vi "Set G08 Delay.vi"(7 "DG Number":i32, 8 "error in (no error)":errorcluster, 11 "Settings":T1={"Channel"=2, "Fire First (µs)"=0.0, "Pulse Width (µs)"=0.005, "Output Modulo"=1, "Output Offset"=0, "Go Signal"=16, "Polarity"=TRUE, "Terminate"=TRUE, "Disconnect (E,F)"=FALSE, "Onto MsBus (E,F)"=FALSE, "Input Positive (E,F)"=TRUE} {"Go Signal" format="%04x" items=["Local Primary"=1, "Local Secondary"=2, "Local Force"=4, "Resynchronize"=8, "Master Primary"=16, "Master Secondary"=32, "Master Force"=64, "System Clock"=128, "Delay Clock"=256, "Inhibit Local"=512, "Start Local"=1024, "Start Bus"=2048, "Step Back Local"=4096, "Step Back Bus"=8192, "From E"=65536, "From F"=131072, "From Bus"=262144]; "Pulse Width (µs)" min=0.0 max=8947840.0 format="%.6f"; "Fire First (µs)" min=0.0 format="%.6f"; "Channel" items=["T"=1, "A"=2, "B"=3, "C"=4, "D"=5, "E"=6, "F"=7]}) -> (0 "error out":errorcluster)   [LabVIEW 2009, in "POLARIS BME DG.lvlib"]
doc: "long Set_BME_G05(double FireFirst_T0, unsigned long OutputModulo_T0, BOOL Active_T0, BOOL Positive_T0, BOOL Terminate_T0, BOOL HighDrive_T0, double FireFirst_A, unsigned long OutputModulo_A, BOOL Active_A, BOOL Positive_A, BOOL Terminate_A, BOOL HighDrive_A, double FireFirst_B, unsigned long OutputModulo_B, BOOL Active_B, BOOL Positive_B, BOOL Terminate_B, BOOL HighDrive_B, BOOL Gate_AB, unsigned long OutputLevel, BOOL TriggerTerminate, BOOL ClockEnable, double InternalClock, double TriggerLevel, unsigned long PresetValue, unsigned long DivideBy, unsigned long ClockSource, unsigned long GateDivider, BOOL PositiveGate, BOOL InternalTrigger, BOOL InternalArm, BOOL SoftwareTrigger, BOOL RisingEdge, BOOL StopOnPreset, BOOL ResetWhenDone, BOOL TriggerEnable, long DG_Number);"
uses:
  POLARIS BME DG.lvlib
  BME DLL/DelayGenerator.dll
panel:
  # "NOTICE -- YOU MUST LEAVE THIS NOTICE IN PLACE.  PER THE TERMS OF THE LICENSE BELOW, YOU MAY SUBLICENSE THIS SOFTWARE \nIN ANY WAY THAT DOES NOT CONFLICT WITH THIS LICENSE.\n\n### BSD License (http://www.opensource.org/licenses/bsd-license.php) Begin ###\n \nCopyright (c) 2011, Applied Energetics, http://www.appliedenergetics.com,\n                               Richard Schwerdtfeger, <rschwerdtfeger@appliedenergetics.com>\n\nAll rights reserved.\n\nRedistribution and use in source and binary forms, with or without modification, are permitted provided that the \nfollowing conditions are met:\n\n    * Redistributions of source code must retain the above copyright notice, this list of conditions and the following disclaimer.\n    * Redistributions in binary form must reproduce the above copyright notice, this list of conditions and the following disclaimer \n       in the documentation and/or other materials provided with the distribution.\n    * Neither the name of Richard Schwerdtfeger, Applied Energetics, Inc., nor the names of its contributors may be used to \n       endorse or promote products derived from this software without specific prior written permission.\n\nTHIS SOFTWARE IS PROVIDED BY THE COPYRIGHT HOLDERS AND CONTRIBUTORS \"AS IS\" AND ANY EXPRESS OR IMPLIED WARRANTIES, \nINCLUDING, BUT NOT LIMITED TO, THE IMPLIED WARRANTIES OF MERCHANTABILITY AND FITNESS FOR A PARTICULAR PURPOSE ARE \nDISCLAIMED. IN NO EVENT SHALL THE COPYRIGHT OWNER OR CONTRIBUTORS BE LIABLE FOR ANY DIRECT, INDIRECT, INCIDENTAL,\n SPECIAL, EXEMPLARY, OR CONSEQUENTIAL DAMAGES (INCLUDING, BUT NOT LIMITED TO, PROCUREMENT OF SUBSTITUTE GOODS OR \nSERVICES; LOSS OF USE, DATA, OR PROFITS; OR BUSINESS INTERRUPTION) HOWEVER CAUSED AND ON ANY THEORY OF LIABILITY, \nWHETHER IN CONTRACT, STRICT LIABILITY, OR TORT (INCLUDING NEGLIGENCE OR OTHERWISE) ARISING IN ANY WAY OUT OF THE USE \nOF THIS SOFTWARE, EVEN IF ADVISED OF THE POSSIBILITY OF SUCH DAMAGE.\n\n### BSD License End ###"
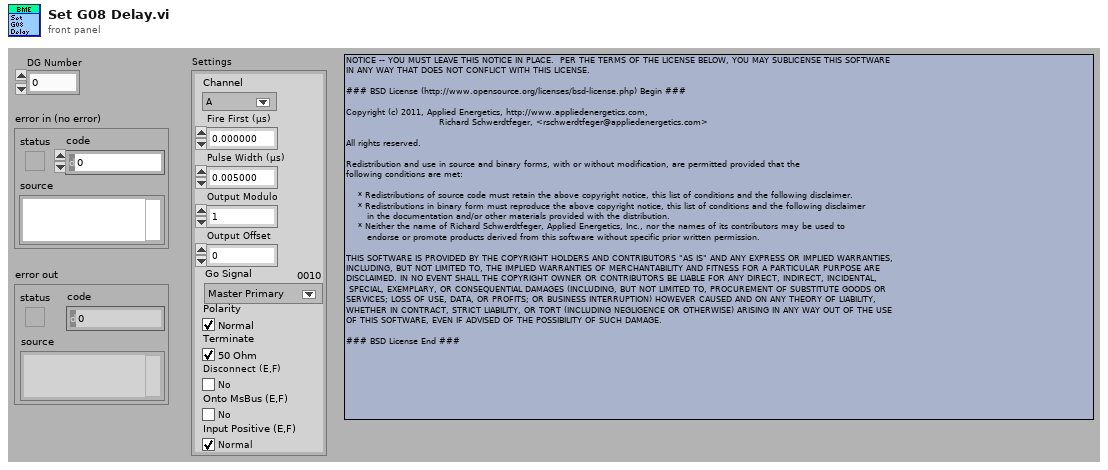
[diagram p1: front panel]
types:
  T1 = cluster{"Channel":u32, "Fire First (µs)":dbl, "Pulse Width (µs)":dbl, "Output Modulo":u32, "Output Offset":u32, "Go Signal":u32, "Polarity":bool, "Terminate":bool, "Disconnect (E,F)":bool, "Onto MsBus (E,F)":bool, "Input Positive (E,F)":bool}
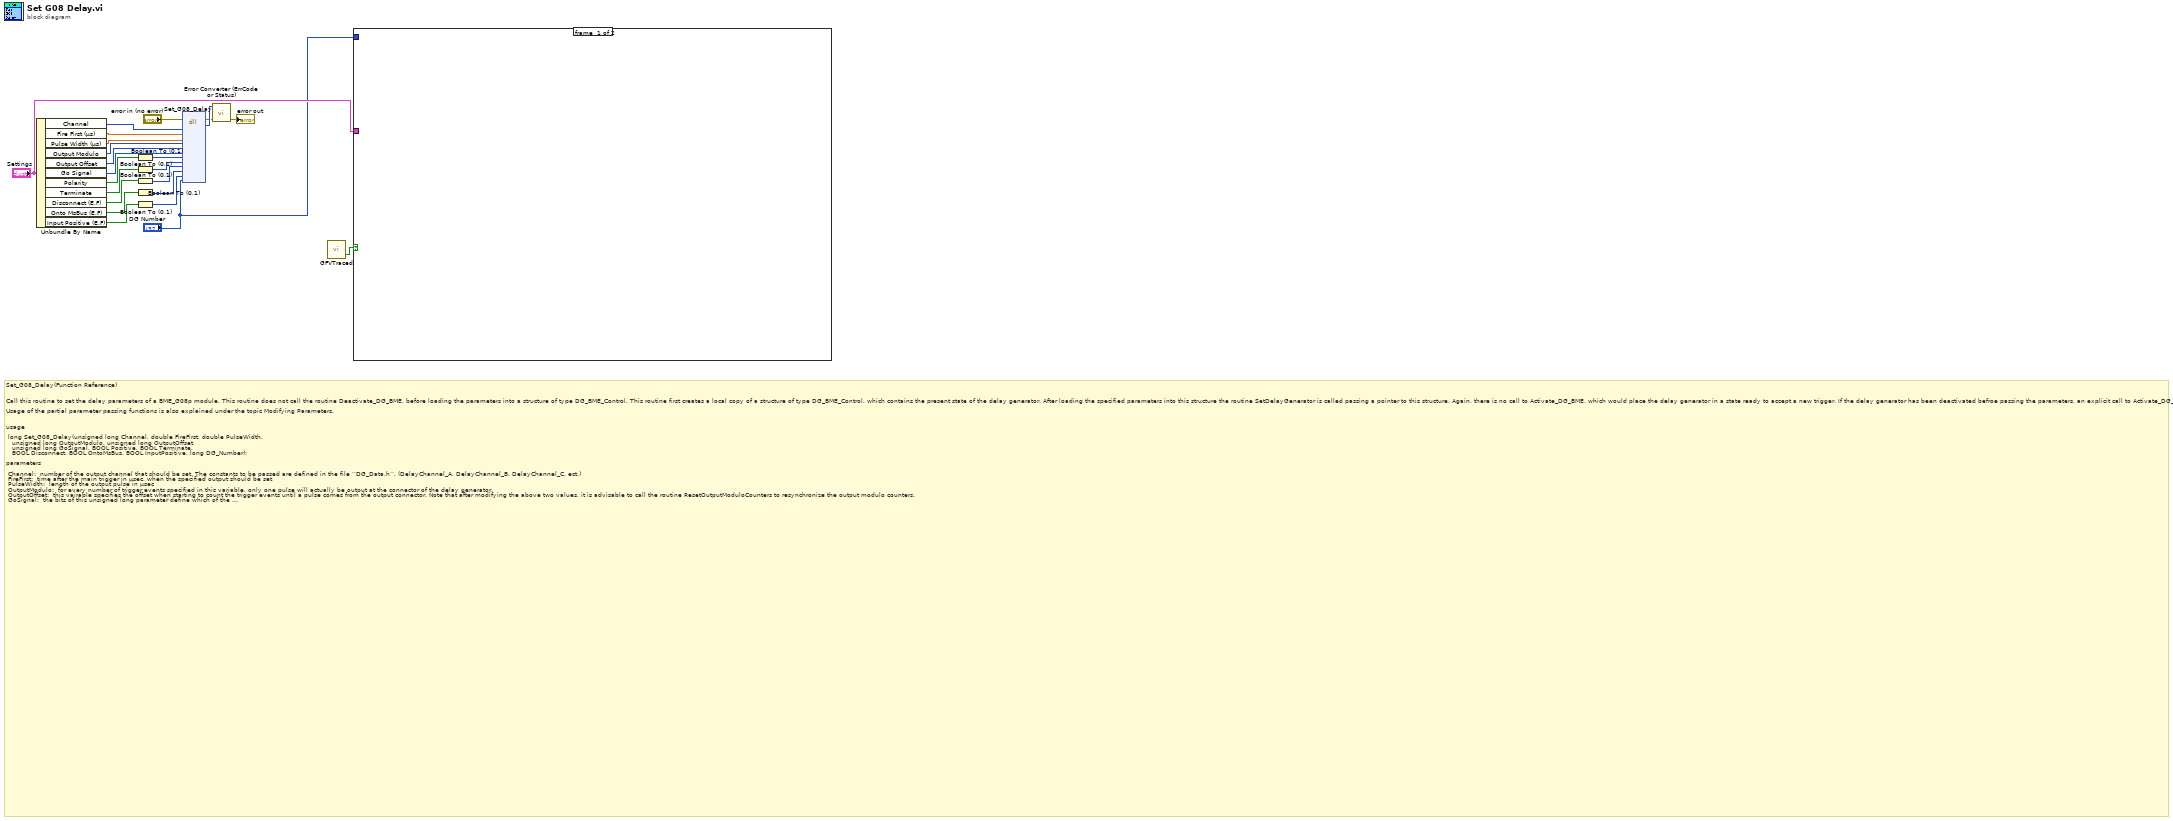
[diagram p0: block diagram]
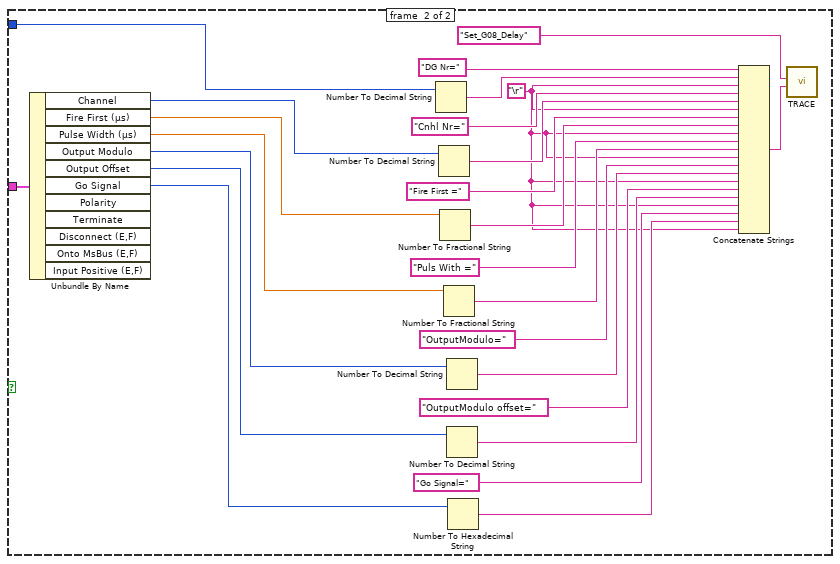
[diagram p2: hidden frame]
diagram:
  # "Set_G08_Delay(Function Reference)\n\n\nCall this routine to set the delay parameters of a BME_G08p module. This routine does not call the routine Deactivate_DG_BME, before loading the parameters into a structure of type DG_BME_Control. This routine first creates a local copy of a structure of type DG_BME_Control, which contains the present state of the delay generator. After loading the specified parameters into this structure the routine SetDelayGenerator is called passing a pointer to this structure. Again, there is no call to Activate_DG_BME, which would place the delay generator in a state ready to accept a new trigger. If the delay generator has been deactivated befroe passing the parameters, an explicit call to Activate_DG_BME is necessary.\n\nUsage of the partial parameter passing functions is also explained under the topic Modifying Parameters.\n\n\nusage\n\n\tlong Set_G08_Delay(unsigned long Channel, double FireFirst, double PulseWidth,\n\t\t\tunsigned long OutputModulo, unsigned long OutputOffset,\n\t\t\tunsigned long GoSignal, BOOL Positive, BOOL Terminate, \n\t\t\tBOOL Disconnect, BOOL OntoMsBus, BOOL InputPositive, long DG_Number);\n\nparameters\n\n\tChannel:\t\tnumber of the output channel that should be set. The constants to be passed are defined in the file ‘’DG_Data.h’’. (DelayChannel_A, DelayChannel_B, DelayChannel_C, ect.)\n\tFireFirst:\t\ttime after the main trigger in µsec, when the specified output should be set\n\tPulseWidth:\t\tlength of the output pulse in µsec\n\tOutputModulo:\t\tfor every number of trigger events specified in this variable, only one pulse will actually be output at the connector of the delay generator.\n\tOutputOffset:\t\tthis vairable specifies the offset when starting to count the trigger events until a pulse comes from the output connector. Note that after modifying the above two values, it is advisable to call the routine ResetOutputModuloCounters to resynchronize the output modulo counters.\n\tGoSignal:\t\tthe bits of this unsigned long parameter define which of the trigger signals available starts this channel. These signals can or’ed. The corresponding constants are defined in ‘’DG_Data.h’’.)\n\t\tLocalPrimary = 0x1:\t\tthe primary trigger signal is used to start the channel.\n\t\tLocalSecondary = 0x2:\t\tthe secondary trigger signal is used to start the channel\n\t\tLocalForce = 0x4: \t\tthe signal from the force trigger counter is used to start the channel.\n\t\tMasterPrimary = 0x10: \t\tthe signal from the master/slave-bus is used to start the channel.\n\t\tSystemClock = 0x80: \t\tthe clock of the delay generator is routed to the output of this channel according to the selection of the DelayClock bit (only possible for the A and B channel of the BME_SG08P)\n\t\tDelayClock = 0x100: \t\tif this bit is set together with the SystemClock, the delay clock of the delay generator is routed to the output of this channel, otherwise the system clock (only possible for the A and B channels) \n\t\tInhibitLocal = 0x200: \t\tthis bit can be set when the clock source selected is TriggerAndOscillator which corresponds to the item trigger->crystal in the Configure Delay Generator dialog window. Setting this bit will inhibit the respective output channel when the local quartz oscillator has taken over after failure of he external clock signal.\n\t\tStartLocal = 0x400: \t\twhen this bit is set, the signal from the local F output connector is used to set the delay lists to their start position.\n\t\tStartBus = 0x800: \t\twhen this bit is set, the signal from the F output connector of the master card is used to set the delay lists to their start position.\n\t\tStepBackLocal = 0x1000: \twhen this bit is set, the signal from the local step back counter is used to step the delay lists back as prescribed by the value in the step back array.\n\t\tStepBackBus = 0x2000: \twhen this bit is set, the signal from the step back counter of the master card is used to step the delay lists back as prescribed by the value in the step back array.\n\t\tEnableFromE = 0x10000: \twhen this bit is set, the delay channel will only produce an output signal when the signal coming from the E output connector is true.\n\t\tEnableFromF = 0x20000: \twhen this bit is set, the delay channel will only produce an output signal when the signal coming from the F output connector is true.\n\t\tEnableFromBus = 0x40000: \twhen this bit is set, the delay channel will only produce an output signal when the signal coming from the master/slave bus is true.\n\tPositive:\t\tTRUE to specify a positive output polarity, otherwise FALSE\n\tTerminate:\t\tTRUE to specify an internal 50 ohm termination on the specified output,otherwise FALSE\n\tDisconnect:\t\tset this flag to TRUE for channels E or F of the BME_SG08 card if the output driver should be disconnected from the connector at the slot. The output driver must be disconnected, if some external signal is to be entered.\n\tOntoMsBus:\t\tset this flag to TRUE for channels E or F of the BME_SG08 card if the signal from this connector should be placed onto the master/slave bus for use at the slave cards\n\tInputPositive:\t\tset this flag to FALSE for channels E or F of the BME_SG08 card if the signal should be inverted before it is used e.g. as enable.\n\tDG_Number:\t\tThe number of the delay generator as assigned by the Initialize_DG_BME routine\n\nreturn value\n\n\t0:  success\n\t2:  DG_Number is out of range\n\t3:  the FireFirst time of an output is negative while the Active flag is TRUE.\n\t5:  one or more delay time(s) is specified too long"
  n1 = Unbundle By Name("Settings") -> ("Channel"=w14:u32, "Fire First (µs)"=w13:dbl, "Pulse Width (µs)"=w12:dbl, "Output Modulo"=w11:u32, "Output Offset"=w10:u32, "Go Signal"=w9:u32, "Polarity"=w19:bool, "Terminate"=w18:bool, "Disconnect (E,F)"=w17:bool, "Onto MsBus (E,F)"=w16:bool, "Input Positive (E,F)"=w15:bool)
  n2 = Boolean To (0,1)(Boolean=w19) -> (0, 1=w8:i16)
  n3 = Boolean To (0,1)(Boolean=w18) -> (0, 1=w7:i16)
  n4 = Boolean To (0,1)(Boolean=w17) -> (0, 1=w6:i16)
  n5 = Boolean To (0,1)(Boolean=w16) -> (0, 1=w5:i16)
  n6 = Boolean To (0,1)(Boolean=w15) -> (0, 1=w4:i16)
  n7 = dll-call lib="D:/CS Framework/LVSCC/LV2009/GPL/Projects/cs-framework/CSClass/CSPOLARIS/POLARIS BME DG/BME DLL/DelayGenerator.*" fn="Set_G08_Delay"(error in="error in (no error)", "Channel"=w14, "FireFirst"=w13, "PulseWidth"=w12, "OutputModulo"=w11, "OutputOffset"=w10, "GoSignal"=w9, "Positive"=w8, "Terminate"=w7, "Disconnect"=w6, "OntoMsBus"=w5, "InputPositive"=w4, "DG_Number"="DG Number") -> (error out=w22:errorcluster, "return type"=w23:i32)  [unwired: 14 in, 1 out]
  n8 = call "Error Converter (ErrCode or Status).vi"("error in (no error)"=w22, "error code"=w23) -> ("error out"=→"error out":errorcluster)  [unwired: 9 out]
  n9 = call "GFVTraced.vi"() -> ("traced?"=w3:bool)  [unwired: 2 in]
  n10 = case shown="True" w3 {
    tunnel: "Settings" -> [_ w45]
    tunnel: "DG Number" -> [_ w24]
    frame #0 {
    }
    frame #1 {
      w25 = "\r"
      n11 = Unbundle By Name(w45) -> ("Channel"=w42:u32, "Fire First (µs)"=w39:dbl, "Pulse Width (µs)"=w35:dbl, "Output Modulo"=w32:u32, "Output Offset"=w29:u32, "Go Signal"=w27:u32)  [unwired: 5 out]
      n12 = Number To Decimal String(number=w24) -> (decimal integer string=w44:string)  [unwired: 1 in]
      n13 = Number To Decimal String(number=w42) -> (decimal integer string=w41:string)  [unwired: 1 in]
      n14 = Number To Fractional String(number=w39) -> (F-format string=w38:string)  [unwired: 3 in]
      n15 = Number To Fractional String(number=w35) -> (F-format string=w36:string)  [unwired: 3 in]
      n16 = Number To Decimal String(number=w32) -> (decimal integer string=w33:string)  [unwired: 1 in]
      n17 = Number To Decimal String(number=w29) -> (decimal integer string=w30:string)  [unwired: 1 in]
      n18 = Number To Hexadecimal String(2:w27) -> (0:w26:string)  [unwired: 1 in]
      n19 = Concatenate Strings("DG Nr=", w44, w25, "Cnhl Nr=", w41, w25, "Fire First =", w38, w25, "Puls With =", w36, w25, "OutputModulo=", w33, w25, "OutputModulo offset=", w30, w25, "Go Signal=", w26, w25) -> (w46:string)
      n20 = call "TRACE.vi"("Parameter String"=w46, "Function"="Set_G08_Delay") -> ()  [unwired: 10 in]
    }
  }
